vi "LVClass_DataServer Start.vi"(0 "DataServer in":refnum<class "DataServer.lvclass">, 11 "error in (no error)":errorcluster) -> (4 "DataServer out":refnum<class "DataServer.lvclass">, 15 "error out":errorcluster)   [LabVIEW 2020, in "DataServer.lvclass"]
doc: "Start server.\n\n<B>serverIn</B> : Pointer to server object.\n<B>serverOut</B> : Pointer to server object."
uses:
  DataServer.lvclass
  DataServer.lvclass/DataServer.ctl
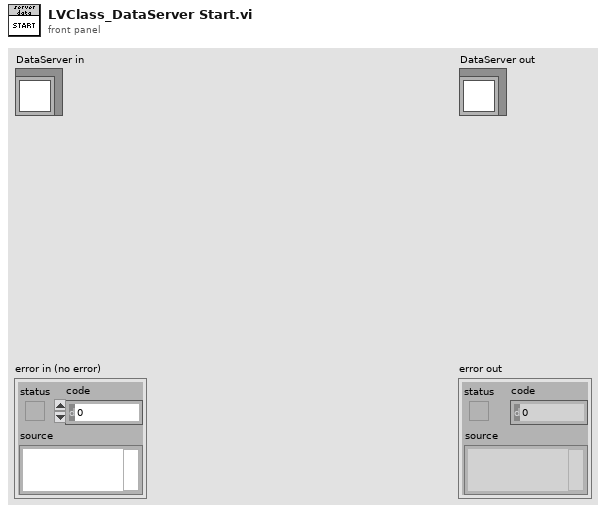
[diagram p1: front panel]
types:
  T1 = typedef "ClassID.ctl" = i64
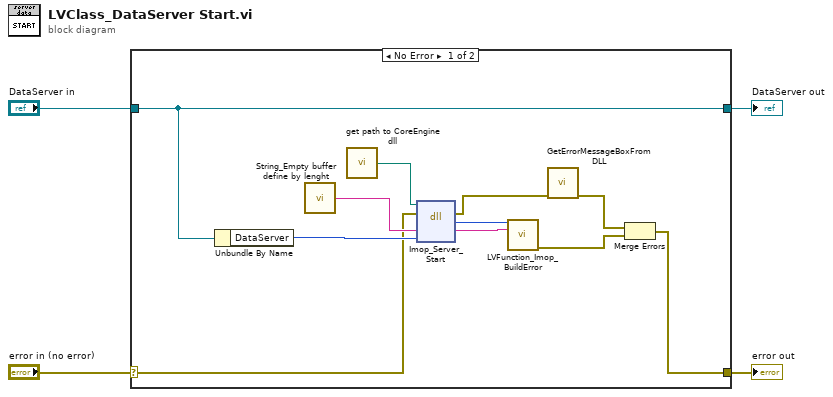
[diagram p0: block diagram]
diagram:
  n1 = case shown="No Error" "error in (no error)" {
    selector: "error in (no error)" -> [w6 w17]
    tunnel: [w5 w17] -> w3
    tunnel: [w7 w16] -> w1
    tunnel: "DataServer in" -> [w7 w16]
    frame No Error {
      n2 = Unbundle By Name(w7) -> ("DataServer"=w13:T1)
      n3 = call "String_Empty buffer define by lenght.vi"() -> ("Empty buffer"=w10:string)  [unwired: 1 in]
      n4 = call "get path to CoreEngine dll.vi"() -> ("path to wavekit library"=w11:path)  [unwired: 14 in, 1 out]
      n5 = dll-call lib="D:/soft/HASO_v3/SVN_trunk/ImOpCoreEngine4_LV2011/DLLs/c_interface_vc100.dll" fn="Imop_Server_Start"(path in=w11, error in=w6, "message"=w10, "server"=w13) -> (error out=w12:errorcluster, "return type"=w8:i32, "message"=w9:string)  [unwired: 2 in, 1 out]
      n6 = call "LVFunction_Imop_BuildError.vi"("code"=w8, "String to Prepend to source (\"\")"=w9) -> ("error out"=w15:errorcluster)  [unwired: 13 in]
      n7 = call "GetErrorMessageBoxFromDLL.vi"("error IN"=w12) -> ("error OUT"=w14:errorcluster)  [unwired: 10 in]
      n8 = Merge Errors(w14, w15) -> (w5:errorcluster)
    }
    frame Error {
    }
  }
  "error out" <- w3
  "DataServer out" <- w1
